vi "TW_Facade.vi"(0 "Data In":T4, 2 "Display State In":T2, 3 "Container State":T3) -> (6 "Data Out":T4, 7 "Display State Out":T2, 8 "Action":T1)   [LabVIEW 2020, in "TW_XControl.xctl"]
uses:
  TW_XControl.xctl
  TW_Data.ctl
  <vilib>/_xctls/Container State.ctl
  TW_State.ctl
  <vilib>/_xctls/Action.ctl
  <vilib>/_xctls/XControlSupport.lvlib
panel:
  out "Toggle":bool
  out "type":string
  out "value":string
  in  "Edit":bool
  in  "Configure":bool
  in  "Property":string
  out "info":string
  in  "Refresh":bool
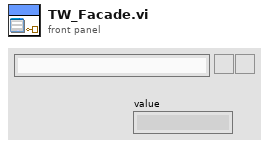
[diagram p1: front panel]
types:
  T1 = typedef "XControlSupport.lvlib/Action.ctl" = cluster{"Data Changed?":bool, "State Changed?":bool, "Action Name":string}
  T2 = typedef "TW_XControl.xctl/TW_State.ctl" = cluster{"Numeric":dbl}
  T3 = typedef "XControlSupport.lvlib/Container State.ctl" = cluster{"Indicator?":bool, "Run Mode?":bool, " Refnum":refnum<vi>}
  T4 = typedef "TW_XControl.xctl/TW_Data.ctl" = string
  T5 = enum8{"Enabled", "Disabled", "Disabled and Grayed Out"}
  T6 = cluster{"Name":string, "BaseURL":string, "AppKey":string, "Headers":string[], "Timeout":i32}
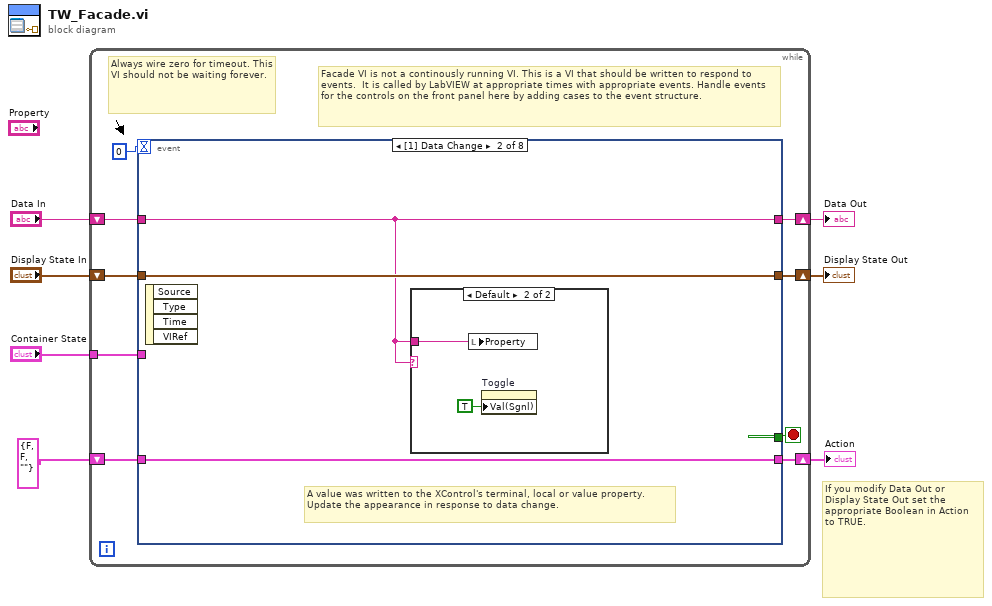
[diagram p0: block diagram]
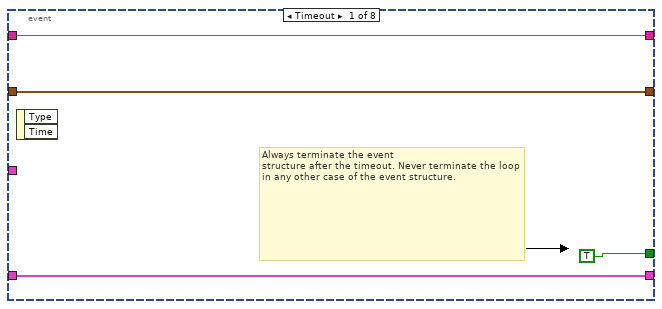
[diagram p2: hidden frame]
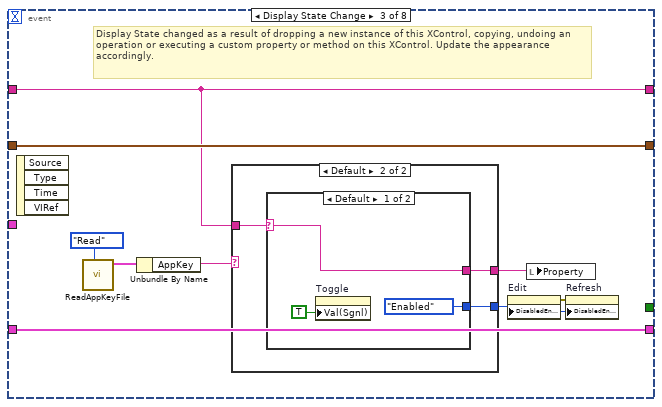
[diagram p4: hidden frame]
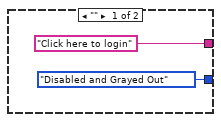
[diagram p5: hidden frame]
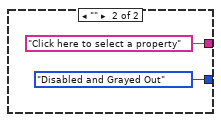
[diagram p6: hidden frame]
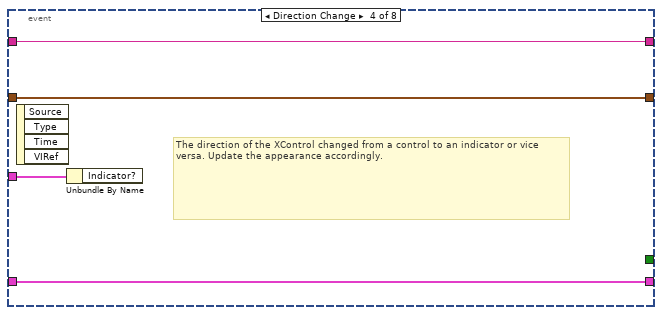
[diagram p7: hidden frame]
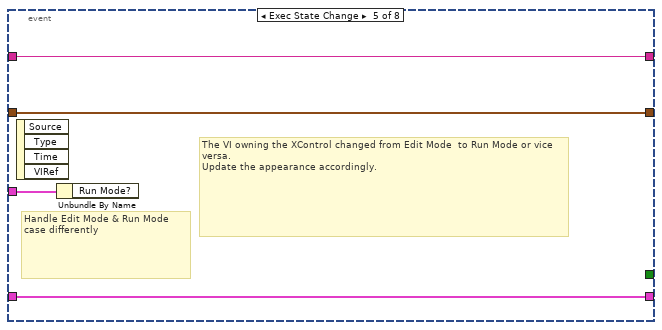
[diagram p8: hidden frame]
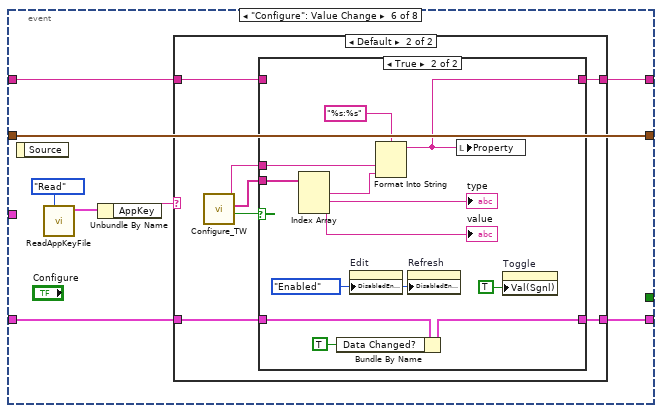
[diagram p9: hidden frame]
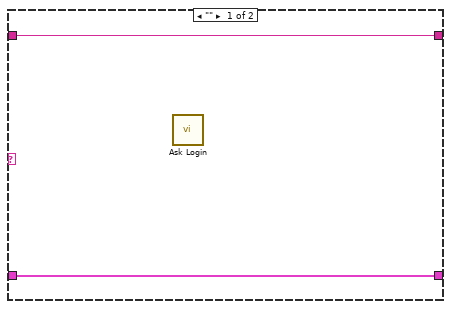
[diagram p10: hidden frame]
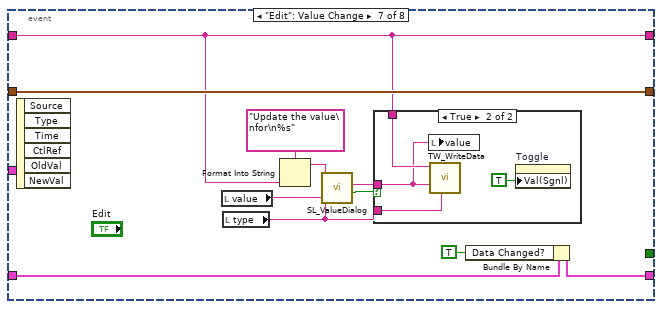
[diagram p12: hidden frame]
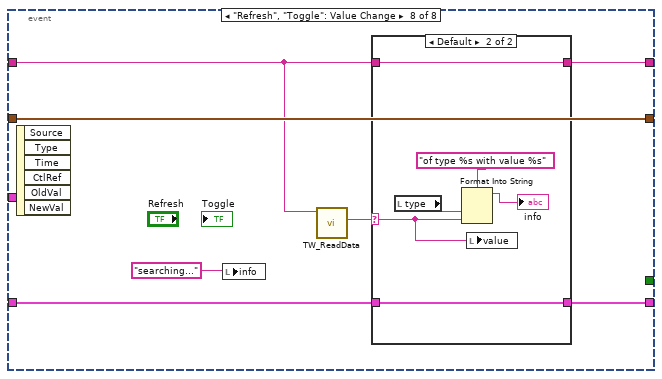
[diagram p14: hidden frame]
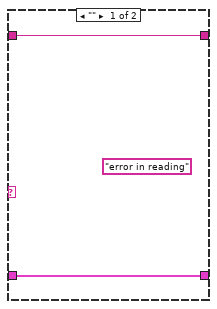
[diagram p15: hidden frame]
diagram:
  # "If you modify Data Out or\nDisplay State Out set the\nappropriate Boolean in Action\nto TRUE."
  n1 = while {
    shift-right: [w15] -> w4
    shift-left: "Display State In" -> [w16]
    tunnel: "Container State" -> [w12]
    shift-right: [w10] -> w7
    shift-left: "Data In" -> [w11]
    shift-right: [w8] -> w2
    shift-left: T1 {"Data Changed?"=FALSE, "State Changed?"=FALSE, "Action Name"=""} ("Action") -> [w9]
    stop <- w14 stop-if-true
    # "Facade VI is not a continously running VI. This is a VI that should be written to respond to events.  It is called by LabVIEW at appropriate times with appropriate events. Handle events for the controls on the front panel here by adding cases to the event structure."
    # "Always wire zero for timeout. This\nVI should not be waiting forever."
    n2 = event shown="[1] Data Change" {
      selector: _ -> [_ _ _ _ _ _ _ _]
      dyn-events: _ -> [_ _ _ _ _ _ _ _]
      timeout: 0 -> [_ _ _ _ _ _ _ _]
      tunnel: w16 -> [w18 w23 w34 w47 w51 w60 w94 w105]
      tunnel: [w18 w23 w34 w47 w51 w60 w94 w105] -> w15
      tunnel: [TRUE _ _ _ _ _ _ _] -> w14
      tunnel: w12 -> [_ _ _ w48 w52 _ _ _]
      tunnel: w11 -> [w17 w21 w28 w46 w50 w59 w85 w100]
      tunnel: [w17 w21 w28 w46 w50 w58 w85 w104] -> w10
      tunnel: [w19 w22 w33 w45 w49 w56 w91 w102] -> w8
      tunnel: w9 -> [w19 w22 w33 w45 w49 w57 w92 w103]
      event Timeout {
        # "Always terminate the event\nstructure after the timeout. Never terminate the loop in any other case of the event structure."
        n3 = event-data() -> ()  [unwired: 1 in, 2 out]
      }
      event Data Change {
        # "A value was written to the XControl's terminal, local or value property.\nUpdate the appearance in response to data change."
        n4 = event-data() -> ()  [unwired: 1 in, 4 out]
        n5 = case shown="Default" w21 {
          tunnel: w21 -> [_ w24]
          frame "" {
          }
          frame Default {
            n6 = local write "Property"(w24) -> ()
            n7 = property on="Toggle" class="Bool (strict)"("Val(Sgnl)"=TRUE ("Value (Signaling)")) -> ()  [unwired: 2 in, 2 out]
          }
        }
      }
      event Display State Change {
        # "Display State changed as a result of dropping a new instance of this XControl, copying, undoing an operation or executing a custom property or method on this XControl. Update the appearance accordingly."
        n8 = event-data() -> ()  [unwired: 1 in, 4 out]
        n9 = call "ReadAppKeyFile.vi"("Task"=enum16{"Read", "Write"}."Read") -> ("Device Out"=w31:T6)  [unwired: 8 in, 2 out]
        n10 = Unbundle By Name(w31) -> ("AppKey"=w30:string)
        n11 = case shown="Default" w30 {
          tunnel: ["Click here to login" ("Property") w39] -> w29
          tunnel: w28 -> [_ w38]
          tunnel: [T5."Disabled and Grayed Out" ("Disabled") w37] -> w26
          frame "" {
          }
          frame Default {
            n12 = case shown="Default" w38 {
              selector: w38 -> [w42 _]
              tunnel: [w42 "Click here to select a property" ("Property")] -> w39
              tunnel: [T5."Enabled" ("Disabled") T5."Disabled and Grayed Out" ("Disabled")] -> w37
              frame Default {
                n13 = property on="Toggle" class="Bool (strict)"("Val(Sgnl)"=TRUE ("Value (Signaling)")) -> ()  [unwired: 2 in, 2 out]
              }
              frame "" {
              }
            }
          }
        }
        n14 = property on="Edit" class="Bool"("DisabledEnum"=w26) -> (error out=w27:errorcluster)  [unwired: 2 in, 1 out]
        n15 = local write "Property"(w29) -> ()
        n16 = property on="Refresh" class="Bool"(error in=w27, "DisabledEnum"=w26) -> ()  [unwired: 1 in, 2 out]
      }
      event Direction Change {
        # "The direction of the XControl changed from a control to an indicator or vice versa. Update the appearance accordingly."
        n17 = event-data() -> ()  [unwired: 1 in, 4 out]
        n18 = Unbundle By Name(w48) -> ()  [unwired: 1 out]
      }
      event Exec State Change {
        # "The VI owning the XControl changed from Edit Mode  to Run Mode or vice versa.\nUpdate the appearance accordingly."
        # "Handle Edit Mode & Run Mode\ncase differently"
        n19 = event-data() -> ()  [unwired: 1 in, 4 out]
        n20 = Unbundle By Name(w52) -> ()  [unwired: 1 out]
      }
      event "Configure": Value Change {
        n21 = event-data() -> ()  [unwired: 1 in, 1 out]
        n22 = call "ReadAppKeyFile.vi"("Task"=enum16{"Read", "Write"}."Read") -> ("Device Out"=w55:T6)  [unwired: 8 in, 2 out]
        n23 = Unbundle By Name(w55) -> ("AppKey"=w53:string)
        n24 = case shown="Default" w53 {
          tunnel: w59 -> [w62 w68]
          tunnel: [w62 w67] -> w58
          tunnel: w57 -> [w61 w64]
          tunnel: [w61 w63] -> w56
          frame "" {
            n25 = call "Ask Login.vi"() -> ()  [unwired: 10 in, 2 out]
          }
          frame Default {
            n26 = call "Configure_TW.vi"() -> ("changed?"=w69:bool, "Property"=w65:string[], "Thing out"=w66:string)  [unwired: 9 in]
            n27 = case shown="True" w69 {
              tunnel: w68 -> [w71 _]
              tunnel: [w71 w76] -> w67
              tunnel: w66 -> [_ w78]
              tunnel: w65 -> [_ w83]
              tunnel: w64 -> [w70 w81]
              tunnel: [w70 w80] -> w63
              frame False {
              }
              frame True {
                w72 = T5."Enabled" ("Disabled")
                n28 = Index Array(array=w83) -> (element #1=w77:string, element #2=→"type":string, element #3=→"value":string)  [unwired: 3 in]
                n29 = Bundle By Name(cluster=w81, "Data Changed?"=TRUE) -> (w80:T1)
                n30 = property on="Edit" class="Bool"("DisabledEnum"=w72) -> ()  [unwired: 2 in, 2 out]
                n31 = Format Into String(format string="%s:%s", w78, w77) -> (resulting string=w76:string)  [unwired: 2 in, 1 out]
                n32 = property on="Refresh" class="Bool"("DisabledEnum"=w72) -> ()  [unwired: 2 in, 2 out]
                n33 = local write "Property"(w76) -> ()
                n34 = property on="Toggle" class="Bool (strict)"("Val(Sgnl)"=TRUE ("Value (Signaling)")) -> ()  [unwired: 2 in, 2 out]
              }
            }
          }
        }
      }
      event "Edit": Value Change {
        n35 = event-data() -> ()  [unwired: 1 in, 6 out]
        n36 = local read "value"() -> (w88:string)
        n37 = local read "type"() -> (w84:string)
        n38 = Format Into String(format string="Update the value\nfor\n%s", w85) -> (resulting string=w89:string)  [unwired: 2 in, 1 out]
        n39 = call "SL_ValueDialog.vi"("type"=w84, "Value"=w88, "Title"=w89) -> ("replace?"=w87:bool, "Value out"=w86:string)  [unwired: 7 in]
        n40 = case shown="True" w87 {
          tunnel: w86 -> [_ w95]
          tunnel: w85 -> [_ w98]
          tunnel: w84 -> [_ w96]
          frame False {
          }
          frame True {
            n41 = local write "value"(w95) -> ()
            n42 = call "TW_WriteData.vi"("Type"=w96, "value"=w95, "Property"=w98) -> ()  [unwired: 9 in]
            n43 = property on="Toggle" class="Bool (strict)"("Val(Sgnl)"=TRUE ("Value (Signaling)")) -> ()  [unwired: 2 in, 2 out]
          }
        }
        n44 = Bundle By Name(cluster=w92, "Data Changed?"=TRUE) -> (w91:T1)
      }
      event "Refresh", "Toggle": Value Change {
        n45 = event-data() -> ()  [unwired: 1 in, 6 out]
        n46 = local write "info"("searching..." ("info")) -> ()
        n47 = call "TW_ReadData.vi"("Property"=w100) -> ("value"=w101:string)  [unwired: 10 in]
        n48 = case shown="Default" w101 {
          selector: w101 -> [_ w108]
          tunnel: w100 -> [w107 w113]
          tunnel: [w107 w113] -> w104
          tunnel: w103 -> [w106 w112]
          tunnel: [w106 w112] -> w102
          frame "" {
            (unwired) "error in reading"
          }
          frame Default {
            n49 = local read "type"() -> (w110:string)
            n50 = Format Into String(format string="of type %s with value %s", w110, w108) -> (resulting string=→"info":string)  [unwired: 2 in, 1 out]
            n51 = local write "value"(w108) -> ()
          }
        }
      }
    }
  }
  "Display State Out" <- w4
  "Data Out" <- w7
  "Action" <- w2
